vi "Create Node.vi"(6 "Parent Index":i32, 8 "Error In":errorcluster, 9 "Folder Path":string, 10 "Project Item":refnum<vi>, 11 "DFS Data In":T1) -> (0 "Error Out":errorcluster, 3 "DFS Data Out":T1)   [LabVIEW 2022 SP3]
doc: "<add documentation here>"
uses:
  DFS Data (cluster).ctl
  DFS Node (cluster).ctl
  DFS Child Node (cluster).ctl
panel:
  # "Development\nControls or indicators that are useful for development or testing, but which are not outputs of the VI."
  # "Input\nInputs to the VI"
  # "Output\nOutputs of the VI"
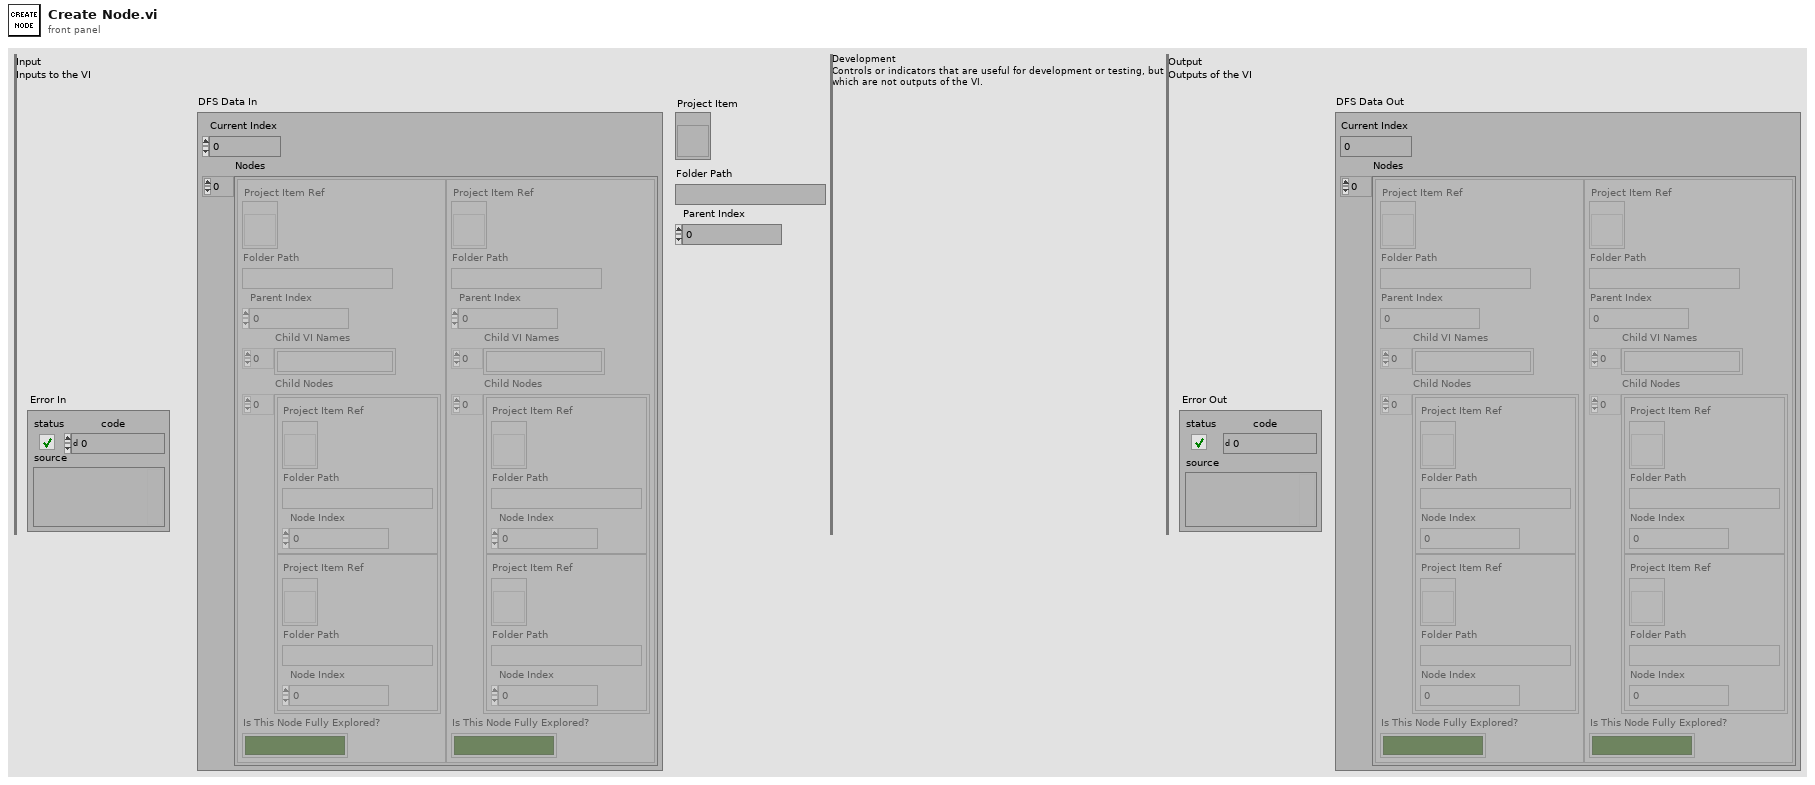
[diagram p1: front panel]
types:
  T1 = typedef "DFS Data (cluster).ctl" = cluster{"Current Index":i32, "Nodes":T2[]}
  T2 = typedef "DFS Node (cluster).ctl" = cluster{"Project Item Ref":refnum<vi>, "Folder Path":string, "Parent Index":i32, "Child VI Names":string[], "Child Nodes":T3[], "Is This Node Fully Explored?":bool}
  T3 = typedef "DFS Child Node (cluster).ctl" = cluster{"Project Item Ref":refnum<vi>, "Folder Path":string, "Node Index":i32}
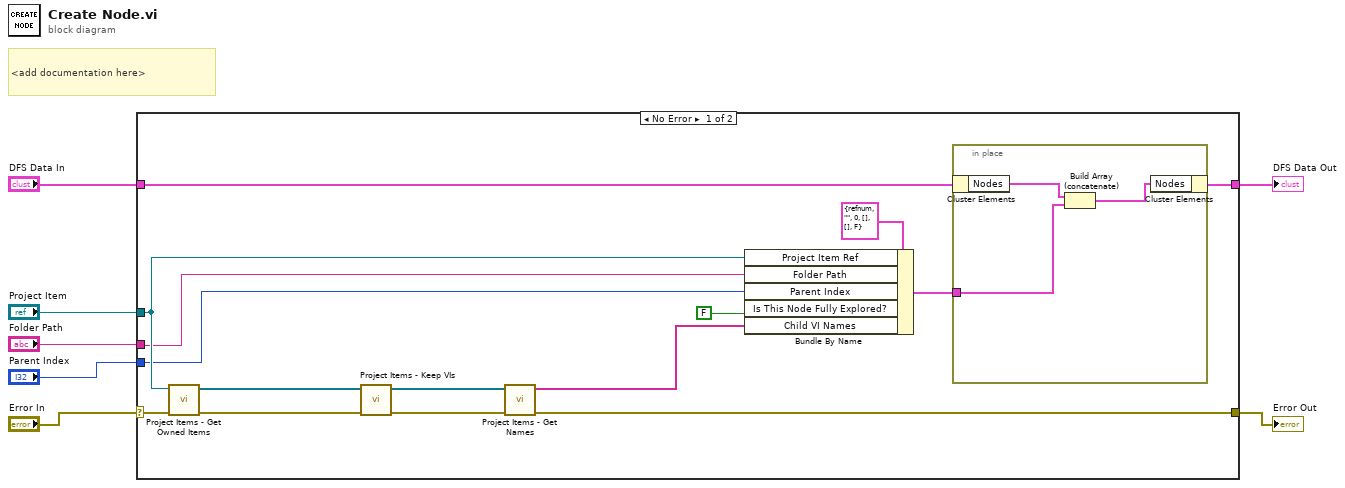
[diagram p0: block diagram]
diagram:
  # "<add documentation here>"
  n1 = case shown="No Error" "Error In" {
    selector: "Error In" -> [w16 w27]
    tunnel: [w11 w27] -> w6
    tunnel: "Project Item" -> [w15 _]
    tunnel: "Folder Path" -> [w12 _]
    tunnel: "Parent Index" -> [w14 _]
    tunnel: "DFS Data In" -> [w10 w26]
    tunnel: [w8 w26] -> w1
    frame No Error {
      n2 = call "Project Items - Get Owned Items.vi"("Error In"=w16, "Project Item"=w15) -> ("Error Out"=w22:errorcluster, "Owned Items"=w13:refnum<vi>[])  [unwired: 8 in]
      n3 = call "Project Items - Keep VIs.vi"("Error In"=w22, "Project Items"=w13) -> ("Error Out"=w19:errorcluster, "Project Items (VIs)"=w20:refnum<vi>[])  [unwired: 8 in]
      n4 = call "Project Items - Get Names.vi"("Error In"=w19, "Project Items"=w20) -> ("Error Out"=w11:errorcluster, "Project Item Names"=w21:string[])  [unwired: 8 in]
      n5 = Bundle By Name(cluster=T2 {"Project Item Ref"=refnum, "Folder Path"="", "Parent Index"=0, "Child VI Names"=[], "Child Nodes"=[], "Is This Node Fully Explored?"=FALSE} ("DFS Data Element"), "Project Item Ref"=w15, "Folder Path"=w12, "Parent Index"=w14, "Is This Node Fully Explored?"=FALSE ("Fully Explored?"), "Child VI Names"=w21) -> (w9:T2)
      n6 = in-place {
        in-place-border: w9 -> [w24]
        n7 = in-place-cluster #1(w10) -> ("Nodes"=w25:T2[])
        n8 = Build Array (concatenate)(w25, w24) -> (w23:T2[])
        n9 = in-place-cluster #1("Nodes"=w23) -> (w8:T1)
      }
    }
    frame Error {
    }
  }
  "Error Out" <- w6
  "DFS Data Out" <- w1
